vi "HeatMap4bin_171213.vi"(8 "Binsize":dbl=4.0, 9 "Array in":dbl[][](array[numeric]), 10 "Y":dbl, 11 "X":dbl) -> (3 "Array out":dbl[][](array[numeric]))   [LabVIEW 2016]
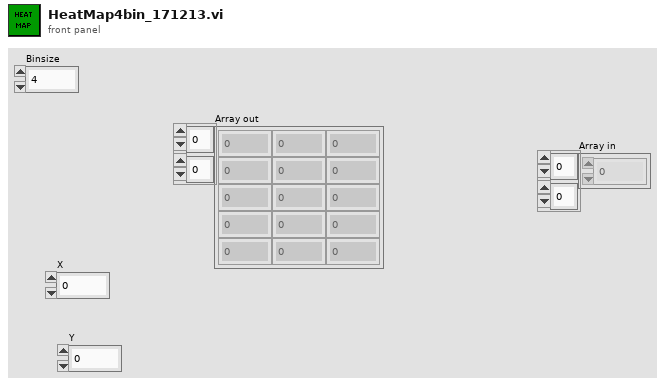
[diagram p1: front panel]
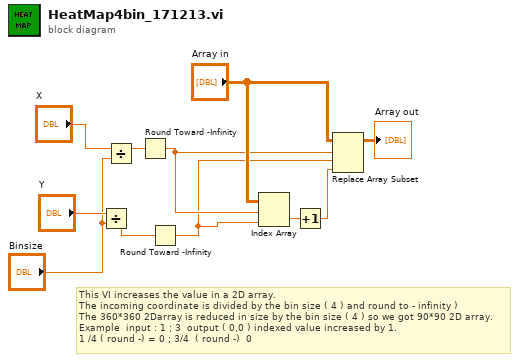
[diagram p0: block diagram]
diagram:
  # "This VI increases the value in a 2D array. \nThe incoming coordinate is divided by the bin size ( 4 ) and round to - infinity ) \nThe 360*360 2Darray is reduced in size by the bin size ( 4 ) so we got 90*90 2D array. \nExample  input : 1 ; 3  output ( 0,0 ) indexed value increased by 1.\n1 /4 ( round -) = 0 ; 3/4  ( round -)  0"
  n1 = Divide(x="Y", y="Binsize") -> (x/y=w4:dbl)
  n2 = Divide(x="X", y="Binsize") -> (x/y=w5:dbl)
  n3 = Round Toward -Infinity(1:w5) -> (0:w3:dbl)
  n4 = Round Toward -Infinity(1:w4) -> (0:w2:dbl)
  n5 = Index Array(array="Array in", index (row)=w3, index (col)=w2) -> (element=w8:dbl)
  n6 = Increment(x=w8) -> (x+1=w9:dbl)
  n7 = Replace Array Subset(array="Array in", new element=w9, index (row)=w3, index (col)=w2) -> (→"Array out":dbl[][])
